vi "test_fgm_partial_pipeline_N22.vi"() -> ()   [LabVIEW 2017, in "MPC_FXP_FGM_TestCase.lvclass"]
uses:
  MPC_FXP_FGM_TestCase.lvclass
  fpga_VIs/fixed-point/typeDefs/x_vec_type.ctl
  fpga_VIs/fixed-point/single-axis/fxp_mpc/fgm_pipiline/quadProgParams_pipe.ctl
  C:/Program Files (x86)/National Instruments/LabVIEW 2017/vi.lib/addons/_JKI Toolkits/VI Tester/TestCase.llb/TestCase.lvclass
  <vilib>/rvi/DesktopExecutionNode/Execution/niFpgaDEN_Execute.vi
  <vilib>/rvi/DesktopExecutionNode/DesktopExecutionNode.xnode
  <userlib>/_VITAC/VITAC.lvlib
panel:
  out "delta u(k)":fxp<+/-,32,3>
  out "error out":errorcluster
  in  "Error In":errorcluster
  out "MPC_FXP_FGM_TestCase.lvclass 2":refnum<class "MPC_FXP_FGM_TestCase.lvclass">
  in  "MPC_FXP_FGM_TestCase.lvclass":refnum<class "MPC_FXP_FGM_TestCase.lvclass">
  out "all rows":dbl[][](array[numeric])
  in  "du_max":fxp<+/-,18,1>=0.197998046875
  out "QP_params":T1={"maxIter"=0, "nuN"=24, "Ns_mpc"=0, "-beta"=-0.9987945556640625, "beta+1"=1.9987945556640625}
  out "z0":dbl[](array[numeric])
  out "y0":dbl[](array[numeric])
  in  "idx2":i16
  out "x_vec":T2=[0.6000000238418579, 0.6000000238418579, -0.5999999940395355, -0.5999999940395355, 0.6000000238418579, 0.6000000238418579, 0.6000000238418579, 0.6000000238418579, -0.5999999940395355, 0.6000000238418579, -0.5999999940395355, -4.0, 0.0, 0.0, 0.0, 0.0, 0.0, 0.0, 0.0, 0.0, 0.0, 0.0, 0.0, 0.0, 0.0]
  out "yi (expected)":fxp<+/-,32,6>[](array[numeric])
  out "zi (expected)":fxp<+/-,32,6>[](array[numeric])
  out "z":fxp<+/-,32,6>[](array[numeric])
  out "y":fxp<+/-,32,6>[](array[numeric])
  in  "xk-COL":i32
  out "idx1-vec":fxp<+/-,32,2>[](array[numeric])
  out "idx2-vec":fxp<+/-,32,2>[](array[numeric])
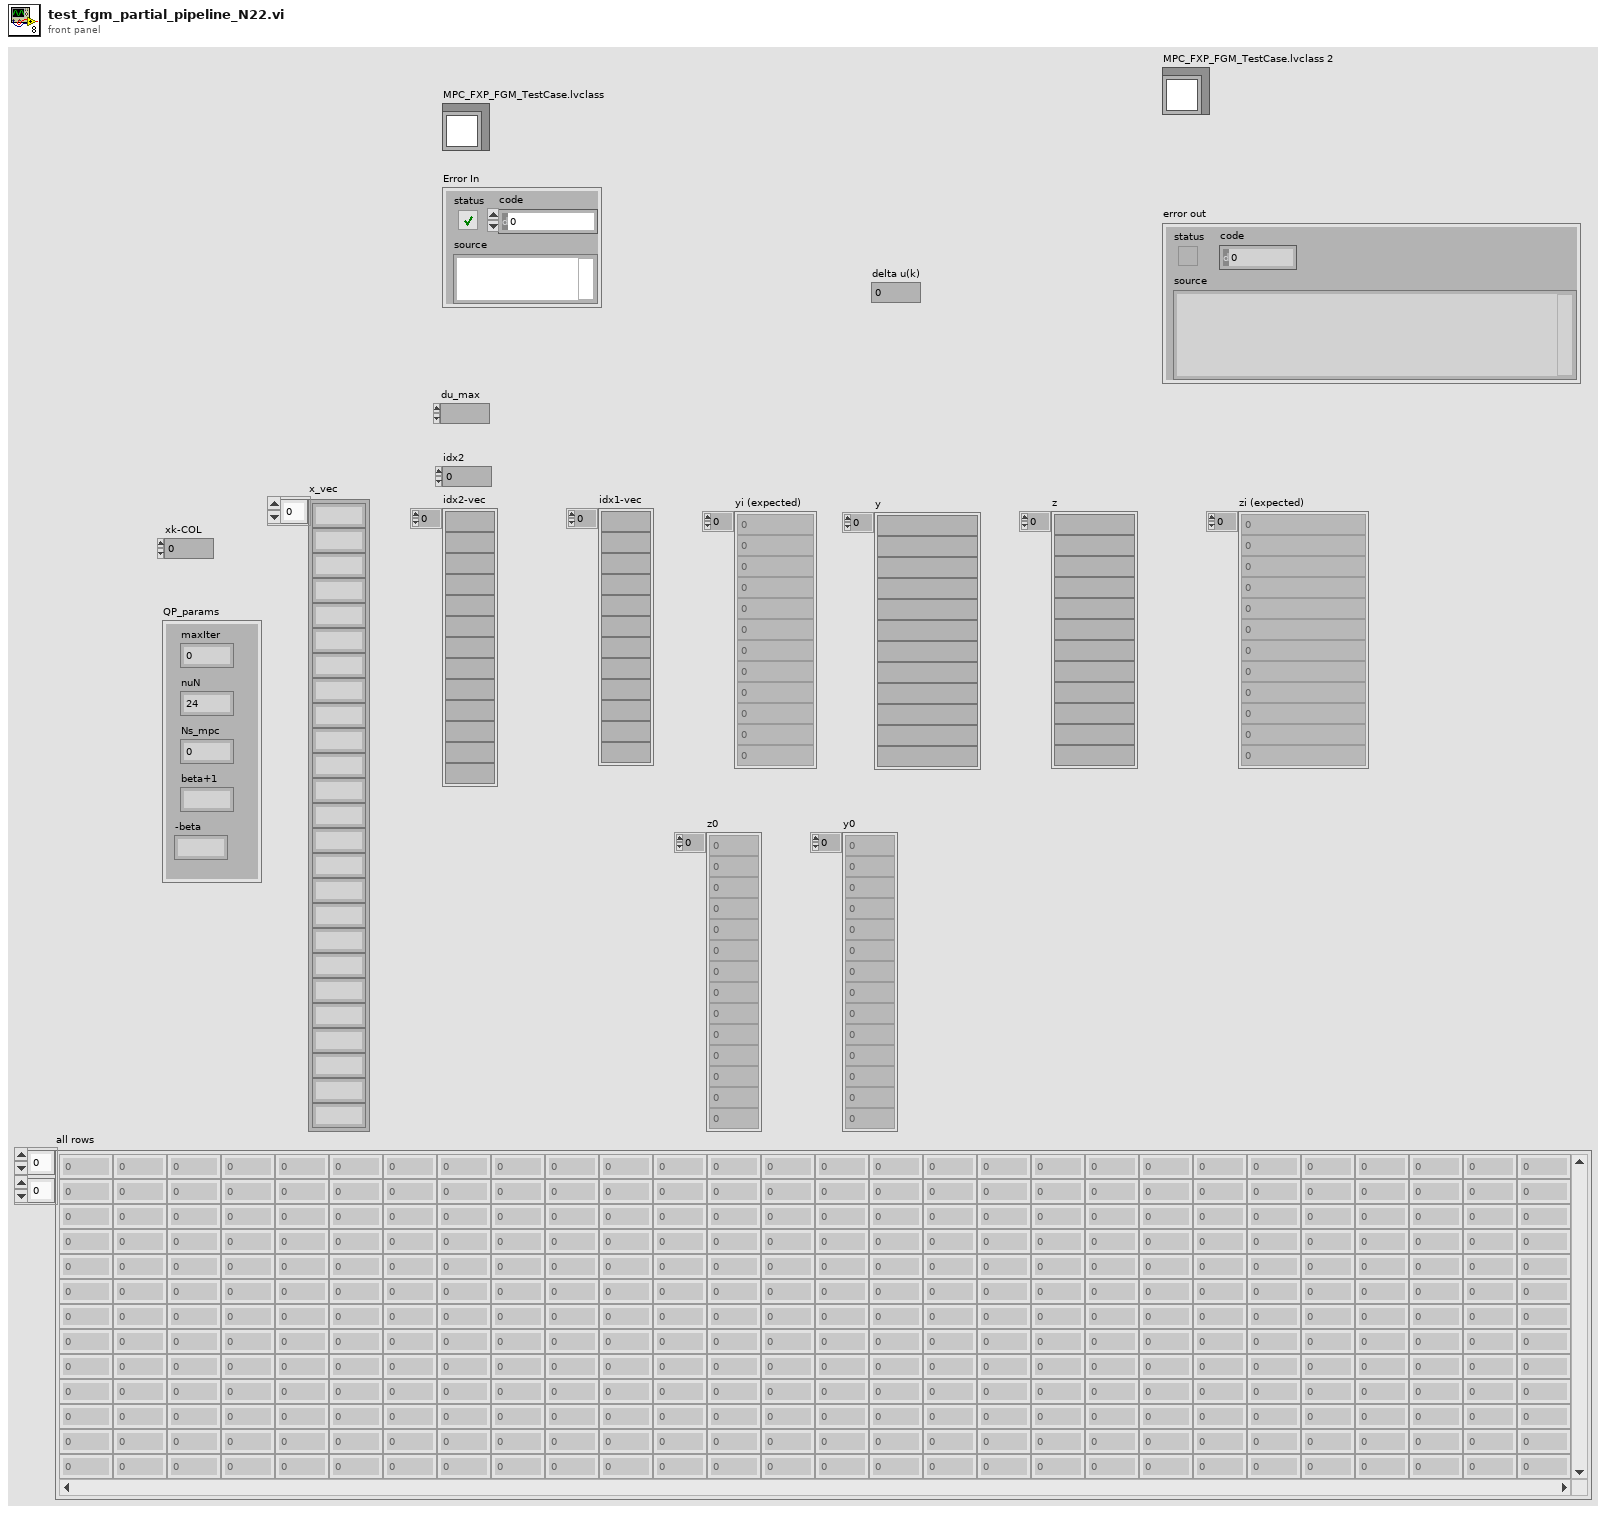
[diagram p1: front panel]
types:
  T1 = typedef "quadProgParams_pipe.ctl" = cluster{"maxIter":u16, "nuN":u16, "Ns_mpc":u16, "-beta":fxp<+/-,18,2>, "beta+1":fxp<+/-,18,2>}
  T2 = typedef "x_vec_type.ctl" = fxp<+/-,32,6>[]
  T3 = typedef "fgm_result_test_data.ctl" = cluster{"z_i_sequence":dbl[][], "y_i_sequence":dbl[][], "X_states":dbl[][]}
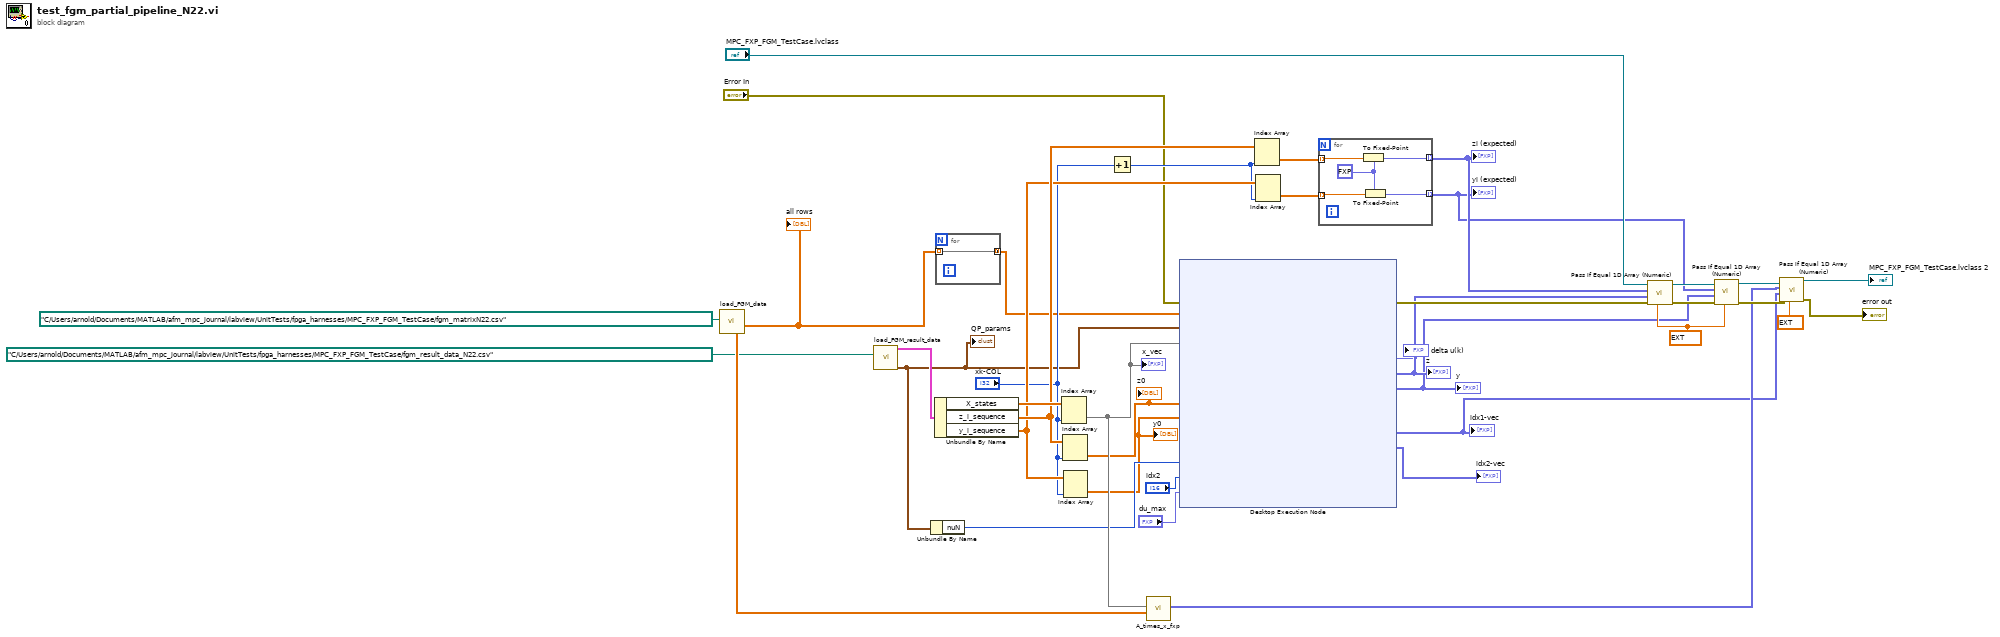
[diagram p0: block diagram]
diagram:
  w23 = ext 0.005 ("delta (optional)")
  n1 = call "load_FGM_data.vi"("Path"=path "C:/Users/arnold/Documents/MATLAB/afm_mpc_journal/labview/UnitTests/fpga_harnesses/MPC_FXP_FGM_TestCase/fgm_matrixN22.csv") -> ("all rows"=w39:dbl[][], "M"=w16:dbl[][])  [unwired: 6 in, 3 out]
  "all rows" <- w39
  n2 = call "load_FGM_result_data.vi"("Path"=path "C:/Users/arnold/Documents/MATLAB/afm_mpc_journal/labview/UnitTests/fpga_harnesses/MPC_FXP_FGM_TestCase/fgm_result_data_N22.csv") -> ("QP_params"=w7:T1, "FGM_result_data"=w38:T3)  [unwired: 8 in, 1 out]
  "QP_params" <- w7
  n3 = Unbundle By Name(w7) -> ("nuN"=w4:u16)
  n4 = Unbundle By Name(w38) -> ("X_states"=w37:dbl[][], "z_i_sequence"=w36:dbl[][], "y_i_sequence"=w35:dbl[][])
  n5 = for {
    tunnel: [w40] -> w8 mode=concatenating
    tunnel: w39 -> [w40] mode=indexing
  }
  n6 = Index Array(array=w37, index (col)="xk-COL") -> (element=w6:dbl[])  [unwired: 1 in]
  "x_vec" <- w6
  n7 = Index Array(array=w36, index (col)="xk-COL") -> (element=w3:dbl[])  [unwired: 1 in]
  "z0" <- w3
  n8 = Index Array(array=w35, index (col)="xk-COL") -> (element=w2:dbl[])  [unwired: 1 in]
  "y0" <- w2
  n9 = Increment(x="xk-COL") -> (x+1=w33:i32)
  n10 = call "A_times_x_fxp.vi"("Az_mat in"=w16, "x_k"=w6) -> ("A*x"=w19:fxp<+/-,64,12>[])  [unwired: 8 in, 1 out]
  n11 = xnode "Desktop Execution Node"("Error In"="Error In", "big_mat_data"=w8, "QP_params"=w7, "x"=w6, "z0"=w3, "y0"=w2, "idx1"=w4, "idx2"="idx2", "du_max"="du_max") -> ("Error Out"=w29:errorcluster, "delta u(k)"=→"delta u(k)":fxp<+/-,32,3>, "z"=w13:fxp<+/-,32,6>[], "y"=w12:fxp<+/-,32,6>[], "idx1"=w11:fxp<+/-,32,6>[], "idx2"=→"idx2-vec":fxp<+/-,32,6>[])
  "idx1-vec" <- w11
  "y" <- w12
  "z" <- w13
  n12 = Index Array(array=w36, index (col)=w33) -> (element=w32:dbl[])  [unwired: 1 in]
  n13 = Index Array(array=w35, index (col)=w33) -> (element=w31:dbl[])  [unwired: 1 in]
  n14 = for {
    tunnel: w32 -> [w45] mode=indexing
    tunnel: w31 -> [w43] mode=indexing
    tunnel: [w44] -> w27 mode=indexing
    tunnel: [w42] -> w24 mode=indexing
    w41 = fxp<+/-,32,6> 0.0 ("fixed-point type")
    n15 = To Fixed-Point(fixed-point type=w41, number=w45) -> (fixed-point=w44:fxp<+/-,32,6>)
    n16 = To Fixed-Point(fixed-point type=w41, number=w43) -> (fixed-point=w42:fxp<+/-,32,6>)
  }
  "zi (expected)" <- w27
  "yi (expected)" <- w24
  n17 = call <userlib>:"Pass If Equal 1D Array (Numeric).vi"("delta (optional)"=w23, "error in (no error)"=w29, "actual"=w13, "expected"=w27, "TestCase in"="MPC_FXP_FGM_TestCase.lvclass") -> ("error out"=w25:errorcluster, "TestCase out"=w26:refnum<class "MPC_FXP_FGM_TestCase.lvclass">)  [unwired: 5 in]
  n18 = call <userlib>:"Pass If Equal 1D Array (Numeric).vi"("delta (optional)"=w23, "error in (no error)"=w25, "actual"=w12, "expected"=w24, "TestCase in"=w26) -> ("error out"=w20:errorcluster, "TestCase out"=w22:refnum<class "MPC_FXP_FGM_TestCase.lvclass">)  [unwired: 5 in]
  n19 = call <userlib>:"Pass If Equal 1D Array (Numeric).vi"("delta (optional)"=ext 0.00001, "error in (no error)"=w20, "actual"=w11, "expected"=w19, "TestCase in"=w22) -> ("error out"=→"error out":errorcluster, "TestCase out"=→"MPC_FXP_FGM_TestCase.lvclass 2":refnum<class "MPC_FXP_FGM_TestCase.lvclass">)  [unwired: 5 in]
